vi "Get Joystick 3.5.vi"() -> (3 "Robot Controls":T1)   [LabVIEW 2015]
uses:
  Robot Controls.ctl
  Global Variables/Refnum Names.vi
  <vilib>/Rock Robotics/WPI/Utilities/WPI_GetSetVariantRefNum.vi
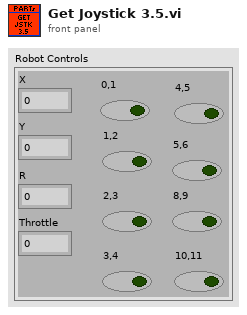
[diagram p1: front panel]
types:
  T1 = typedef "Robot Controls.ctl" = cluster{"X":dbl, "Y":dbl, "R":dbl, "Throttle":dbl, "0,1":bool, "1,2":bool, "2,3":bool, "3,4":bool, "4,5":bool, "5,6":bool, "8,9":bool, "10,11":bool}
  T2 = typedef "WPI_JoystickDevRef.ctl" = cluster{"Device":T3}
  T3 = typedef "WPI_JoystickDeviceEnum.ctl" = enum16{"USB 0", "USB 1", "USB 2", "USB 3", "USB 4", "USB 5"}
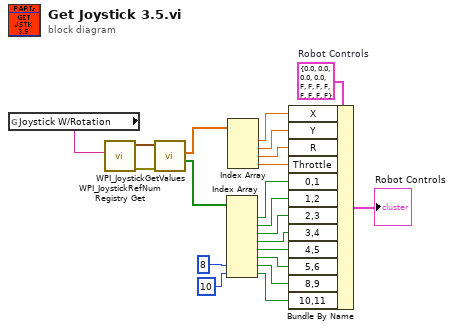
[diagram p0: block diagram]
diagram:
  w2 = T1 {"X"=0.0, "Y"=0.0, "R"=0.0, "Throttle"=0.0, "0,1"=FALSE, "1,2"=FALSE, "2,3"=FALSE, "3,4"=FALSE, "4,5"=FALSE, "5,6"=FALSE, "8,9"=FALSE, "10,11"=FALSE}  # Robot Controls
  n1 = global read "Refnum Names.vi" "Joystick W/Rotation"() -> (w3:string)
  n2 = call <vilib>:"WPI_JoystickRefNum Registry Get.vi"("refnum name"=w3) -> ("error out"=w4:errorcluster, "JoystickDevRef"=w5:T2)  [unwired: 9 in]
  n3 = call <vilib>:"WPI_JoystickGetValues.vi"("error in (no error)"=w4, "JoystickDevRef"=w5) -> ("Buttons"=w7:bool[], "Axes"=w6:dbl[])  [unwired: 5 in, 3 out]
  n4 = Index Array(array=w7, index #7=8 ("index"), index #8=10 ("index")) -> (element #1=w12:bool, element #2=w13:bool, element #3=w14:bool, element #4=w15:bool, element #5=w16:bool, element #6=w17:bool, element #7=w18:bool, element #8=w19:bool)  [unwired: 6 in]
  n5 = Index Array(array=w6) -> (element #1=w8:dbl, element #2=w9:dbl, element #3=w10:dbl, element #4=w11:dbl)  [unwired: 4 in]
  n6 = Bundle By Name(cluster=w2, "X"=w8, "Y"=w9, "R"=w10, "Throttle"=w11, "0,1"=w12, "1,2"=w13, "2,3"=w14, "3,4"=w15, "4,5"=w16, "5,6"=w17, "8,9"=w18, "10,11"=w19) -> (→"Robot Controls":T1)
